vi "velocity_test.vi"() -> ()   [LabVIEW 2018]
uses:
  <vilib>/Platform/TimedLoop/XDataNode/timing_clust.ctl
  <vilib>/Platform/TimedLoop/XDataNode/nitl_modes.ctl
  <vilib>/Platform/TimedLoop/XDataNode/wakeup.ctl
  <vilib>/Platform/TimedLoop/XDataNode/XDataNode.xnode
  <vilib>/Platform/TimedLoop/XDataNode/XDNodeRunTimeDep.lvlib
panel:
  out "Waveform Chart 4":cluster{"V":dbl, "avg.":dbl}(graph)
  in  "no. moving avg. Z":u8=1
  in  "Period":i64=100
  out "Finished Late? [i-1]":bool
  in  "Stop Button":bool
  out "Waveform Chart 2":dbl(graph)
  out "velocity":dbl
  in  "offset (mV)":dbl=-0.04000000000000001
  in  "amplitude (V)":dbl=0.9
  in  "frequency (Hz)":dbl=25.0
  out "avg loop rate":dbl=4.866229289447348
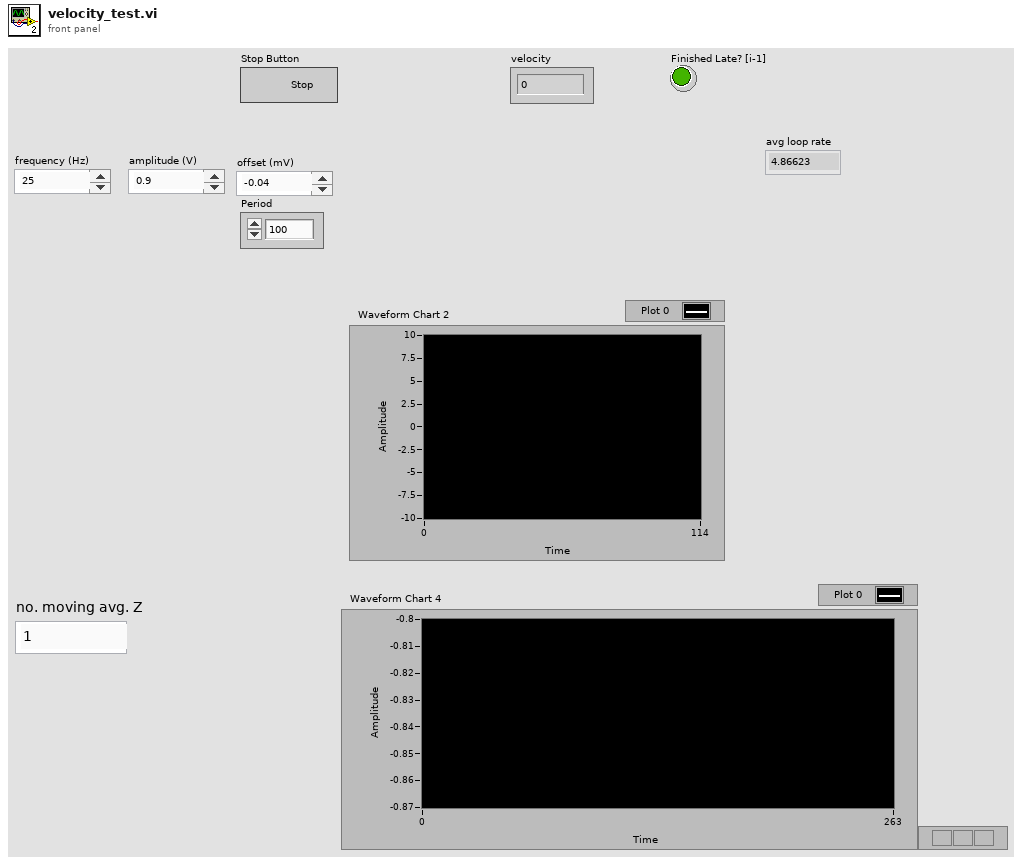
[diagram p1: front panel]
types:
  T1 = typedef "XDNodeRunTimeDep.lvlib/timing_clust.ctl" = cluster{"Expected End [f-1]":u64, "Actual End [f-1]":u64, "Finished Late? [f-1]":bool, "Expected End [i-1]":u64, "Actual End [i-1]":u64, "Finished Late? [i-1]":bool, "Expected Start [i]":u64, "Actual Start [i]":u64, "Expected Start [f]":u64, "Actual Start [f]":u64, "Source Name":string, "Structure Name":string, "Period":i64, "Deadline":i64, "Offset":i64, "Start":i64, "Priority":i32, "Timeout":i32, "Mode":T2, "Wakeup Reason":T3, "Error":errorcluster, "Source Type":string, "Secondary Source Type":string, "Global End Time":u64, "Global Start Time":u64, "Frame Duration":u64, "Iteration Duration":u64, "Assigned CPU":i32, "I/O Scan Engine Mode":u32}
  T2 = typedef "XDNodeRunTimeDep.lvlib/nitl_modes.ctl" = enum32{"No Change", "Process missed periods, maintain original phase", "Discard missed periods, maintain original phase", "Process missed periods, ignore original phase", "Discard missed periods, ignore original phase"}
  T3 = typedef "XDNodeRunTimeDep.lvlib/wakeup.ctl" = enum32{"Normal", "Aborted", "Asynchronous wakeup", "Timing source error", "Timed loop error", "Timeout"}
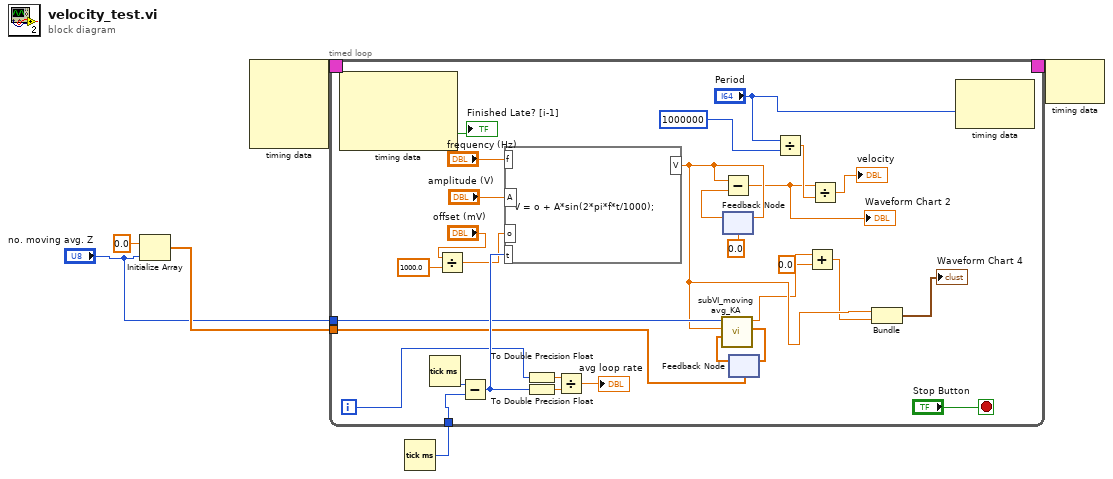
[diagram p0: block diagram]
diagram:
  n1 = Initialize Array(0.0 ("element"), "no. moving avg. Z") -> (w2:dbl[])
  n2 = node-c288() -> (w6:T1)  [unwired: 4 in]
  n3 = Tick Count (ms)() -> (millisecond timer value=w4:u32)
  n4 = timed-loop {
    timing: w6 -> [_]
    timing-out: [_] -> w5
    tunnel: w4 -> [w26]
    tunnel: w2 -> [w14]
    tunnel: "no. moving avg. Z" -> [w13]
    i -> [w25]
    stop <- "Stop Button" stop-if-true
    n5 = node-c288() -> (→"Finished Late? [i-1]":bool)  [unwired: 1 in, 3 out]
    n6 = Tick Count (ms)() -> (millisecond timer value=w36:u32)
    n7 = Divide(x="offset (mV)", y=1000.0) -> (x/y=w27:dbl)
    n8 = Subtract(x=w36, y=w26) -> (x-y=w30:u32)
    n9 = formula code="V = o + A*sin(2*pi*f*t/1000);"("f"="frequency (Hz)", "A"="amplitude (V)", "t"=w30, "o"=w27) -> ("V"=w12:dbl)
    n10 = To Double Precision Float(number=w25) -> (double precision float=w34:dbl)
    n11 = To Double Precision Float(number=w30) -> (double precision float=w35:dbl)
    n12 = Divide(x=w34, y=w35) -> (x/y=→"avg loop rate":dbl)
    n13 = feedback-in #1(w12) -> ()
    n14 = feedback #1(0.0) -> (w24:dbl)
    n15 = Subtract(x=w12, y=w24) -> (x-y=w7:dbl)
    "Waveform Chart 2" <- w7
    n16 = feedback #2(w14) -> (w15:dbl[])
    n17 = call "subVI_moving avg_KA.vi"("input array"=w15, "sample"=w12, "no. moving avg."=w13) -> ("output array"=w16:dbl[], "avg."=w10:dbl)  [unwired: 7 in]
    n18 = feedback-in #2(w16) -> ()
    n19 = Divide(x="Period", y=i64 1000000) -> (x/y=w21:dbl)
    n20 = Add(x=w10, y=0.0) -> (x+y=w8:dbl)
    n21 = Divide(x=w7, y=w21) -> (x/y=→"velocity":dbl)
    n22 = Bundle("V"=w12, w8) -> (→"Waveform Chart 4":cluster{"V":dbl, dbl})  [unwired: 1 in]
    n23 = node-c288("Period") -> ()  [unwired: 1 in, 1 out]
  }
  n24 = node-c288(w5) -> ()  [unwired: 1 out]
